vi "Update from Left.vi"(9 "Col":i32, 10 "Row":i32, 11 "Proto in":refnum<class "Heat Map.lvclass">) -> (3 "Proto out":refnum<class "Heat Map.lvclass">)   [LabVIEW 2021, in "Heat Map.lvclass"]
uses:
  Heat Map.lvclass
  Heat Map.lvclass/Heat Map.ctl
  Direction.ctl
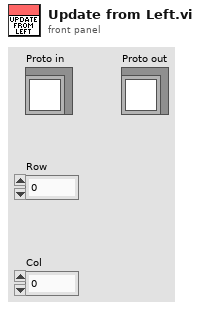
[diagram p1: front panel]
types:
  T1 = typedef "Heat Map.lvclass/Direction.ctl" = enum16{"Up", "Down", "Right", "Left"}
  T2 = map{cluster{"Row":i32, "Col":i32}, set{cluster{"Heat":i32, "Prev Steps":T1[]}}}
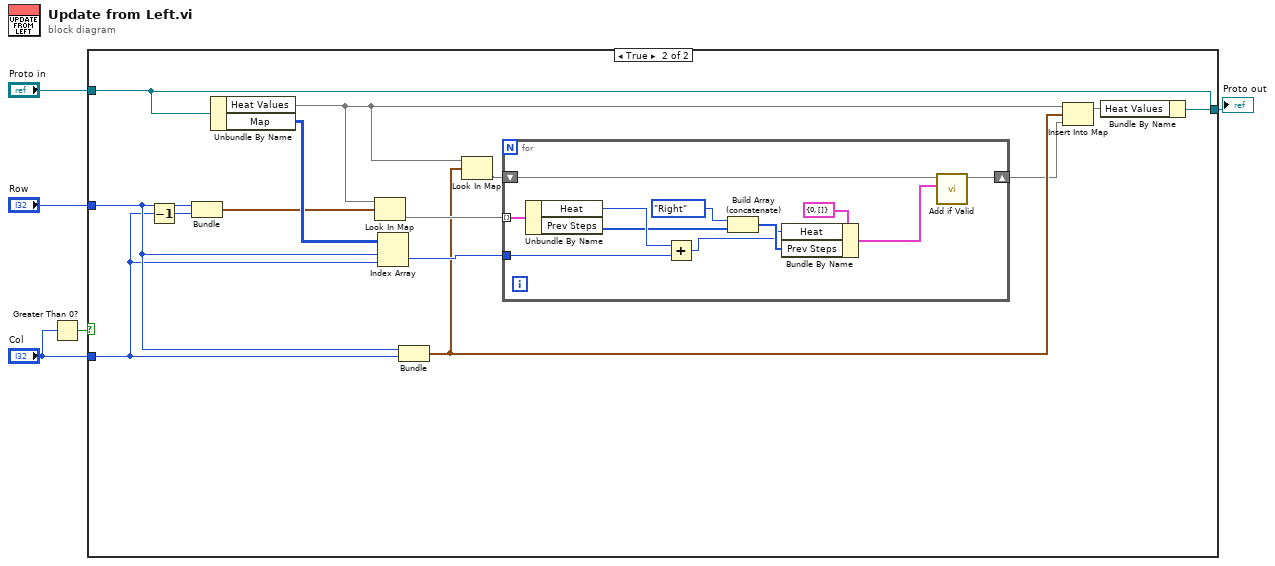
[diagram p0: block diagram]
diagram:
  n1 = Greater Than 0?(x="Col") -> (x > 0?=w1:bool)
  n2 = case shown="True" w1 {
    tunnel: [w6 w18] -> w5
    tunnel: "Proto in" -> [w6 w17]
    tunnel: "Row" -> [_ w13]
    tunnel: "Col" -> [_ w12]
    frame False {
    }
    frame True {
      n3 = Decrement(x=w12) -> (x-1=w11:i32)
      n4 = Bundle("Row"=w13, w11) -> (w16:cluster{"Row":i32, i32})  [unwired: 1 in]
      n5 = Unbundle By Name(w17) -> ("Heat Values"=w10:T2, "Map"=w20:i32[][])
      n6 = Look In Map(map=w10, key=w16) -> (value=w14:set{cluster{"Heat":i32, "Prev Steps":T1[]}})  [unwired: 1 in, 1 out]
      n7 = Index Array(array=w20, index (row)=w13, index (col)=w12) -> (element=w15:i32)
      n8 = Bundle("Row"=w13, "Col"=w12) -> (w9:cluster{"Row":i32, "Col":i32})  [unwired: 1 in]
      n9 = Look In Map(map=w10, key=w9) -> (value=w8:set{cluster{"Heat":i32, "Prev Steps":T1[]}})  [unwired: 1 in, 1 out]
      n10 = for {
        tunnel: w14 -> [w22] mode=indexing
        tunnel: w15 -> [w30]
        shift-right: [w24] -> w7
        shift-left: w8 -> [w25]
        n11 = Unbundle By Name(w22) -> ("Heat"=w31:i32, "Prev Steps"=w29:T1[])
        n12 = Add(x=w31, y=w30) -> (x+y=w26:i32)
        n13 = Build Array (concatenate)(Direction."Right" ("Dir"), w29) -> (w27:T1[])
        n14 = Bundle By Name(cluster=cluster{"Heat":i32, "Prev Steps":T1[]} {"Heat"=0, "Prev Steps"=[]} ("element"), "Heat"=w26, "Prev Steps"=w27) -> (w21:cluster{"Heat":i32, "Prev Steps":T1[]})
        n15 = call "Add if Valid.vi"("element"=w21, "set in"=w25) -> ("set out"=w24:set{cluster{"Heat":i32, "Prev Steps":T1[]}})  [unwired: 9 in]
      }
      n16 = Insert Into Map(map in=w10, key=w9, value=w7) -> (map out=w19:T2)  [unwired: 2 out]
      n17 = Bundle By Name(cluster=w17, "Heat Values"=w19) -> (w18:refnum<class "Heat Map.lvclass">)
    }
  }
  "Proto out" <- w5
